vi "Timer_FGV_main.vi"(7 "Timer Inputs":T2, 8 "Error In":errorcluster) -> (0 "Error Out":errorcluster, 2 "Timer Outputs":T1)   [LabVIEW 2013]
doc: "This functional global variable (FGV) acts as a timer for the SVM burner test VI. It accepts a target time and\nstatus Booleans as arguments, and returns status Booleans and elapsed time indicating whether the flame\nhas been relit, has been lit for long enough, or has blown out.\nArgs:\n Target time (float): target time in seconds for the VI to wait before accepting a flame as stable\n relight? (bool): indicates when we are relighting the flame (do not indicate that flame has blown out)\n flame? (bool): indicates when a flame is detected and the timer should count\n\nReturns:\n Elapsed time (float): time elapsed since the flame became lit. Resets if the flame goes off.\n target reached? (bool): indicates when the flame has been lit for the target duration.\n flame out? (bool): indicates when the flame has blown out. Will not turn True unless relight? is False.\n flame lit? (bool): indicates when the flame has been lit. Will not turn True unless relight? is True."
uses:
  Controls/timer_input_cluster.ctl
  Controls/timer_output_cluster.ctl
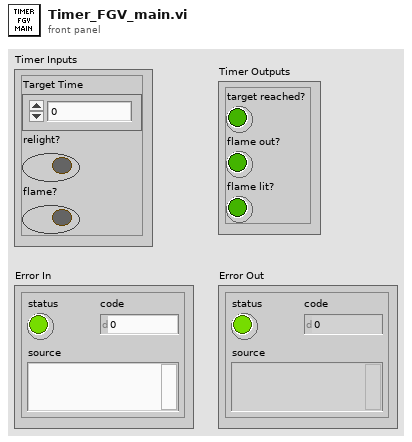
[diagram p1: front panel]
types:
  T1 = typedef "timer_output_cluster.ctl" = cluster{"target reached?":bool, "flame out?":bool, "flame lit?":bool}
  T2 = typedef "timer_input_cluster.ctl" = cluster{"Target Time":dbl, "relight?":bool, "flame?":bool}
  T3 = typedef "timer_state_cluster.ctl" = cluster{"Time Stamp":dbl, "Elapsed Time":dbl}
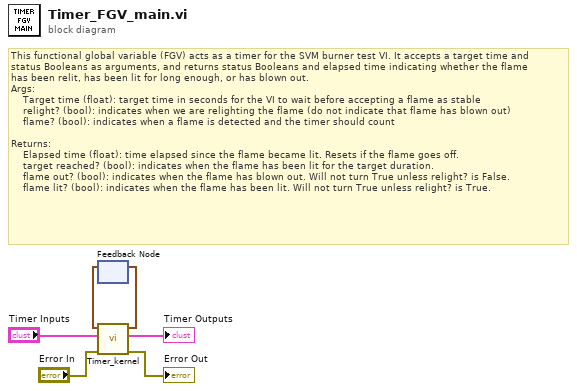
[diagram p0: block diagram]
diagram:
  # "This functional global variable (FGV) acts as a timer for the SVM burner test VI. It accepts a target time and\nstatus Booleans as arguments, and returns status Booleans and elapsed time indicating whether the flame\nhas been relit, has been lit for long enough, or has blown out.\nArgs:\n    Target time (float): target time in seconds for the VI to wait before accepting a flame as stable\n    relight? (bool): indicates when we are relighting the flame (do not indicate that flame has blown out)\n    flame? (bool): indicates when a flame is detected and the timer should count\n\nReturns:\n    Elapsed time (float): time elapsed since the flame became lit. Resets if the flame goes off.\n    target reached? (bool): indicates when the flame has been lit for the target duration.\n    flame out? (bool): indicates when the flame has blown out. Will not turn True unless relight? is False.\n    flame lit? (bool): indicates when the flame has been lit. Will not turn True unless relight? is True."
  n1 = feedback #1() -> (w5:T3)  [unwired: 1 in]
  n2 = call "Timer_kernel.vi"("Error In"="Error In", "Timer Inputs"="Timer Inputs", "Timer States"=w5) -> ("Error Out"=→"Error Out":errorcluster, "Timer Outputs"=→"Timer Outputs":T1, "Timer States out"=w6:T3)  [unwired: 6 in]
  n3 = feedback-in #1(w6) -> ()
